vi "Protocole_son_preparatoire_2020.vi"() -> ()   [LabVIEW 2020]
uses:
  8c73e72c-2e4b-4090-9b5f-4dd0fd0f2149.vi
  bfbeb452-2a3a-4e65-bf29-1a1bdd43f38b.vi
  3aaf8e9c-9ac4-4c40-bc9e-b7ffdc0d35df.vi
  <vilib>/numeric/Random Number (Range) DBL.vi
  0129e9be-af5f-4d34-b4ce-d6aa148f68f5.vi
  2e48d409-a5b3-4865-bc36-115429370ffe.vi
  <vilib>/Analysis/1siggen.llb/General Gauss-Mod Sine.vi
  <vilib>/Analysis/NI_AALBase.lvlib
  <vilib>/measure/NI_MABase.lvlib
panel:
  in  "Control temps bruit 2":cluster{"Fs":dbl, "#s":dbl}={"Fs"=1000.0, "#s"=1000.0} {"Fs" format="%.2p"}
  in  "Control temps bruit":cluster{"Fs":dbl, "#s":dbl}={"Fs"=1000.0, "#s"=1000.0} {"Fs" format="%.2p"}
  in  "Nom du fichier":string="Test_"
  out "Barre de progression":dbl(slide) scale=0.0..100.0
  in  "?":enum32{"Temps", "Numérique "}(tab)
  in  "Temps d'attente entre chaque sons /s":dbl=2.0
  in  "Plus ou moins /s":dbl=1.0
  in  "Différence entre chaque fréquence /Hz":dbl=100.0
  in  "Fréquence min /Hz":dbl=440.0
  in  "Nombre de répétition d'opération":dbl=1.0
  in  "Nombre de sons":dbl=3.0
  in  "Amplitude min /V":dbl=0.5
  in  "Différence entre chaque amplitude /V":dbl=0.2
  in  "Lieu du fichier":path=path "D:/Labview/Stage/LabVIEW 2020/Programmes_utilisables/Protocoles_enregistrement_ampli/Protocole_son_preparatoire_2020/Donnees" caption="Filename"
  in  "?":bool
  # "Pas touché"
  # "Protocole :"
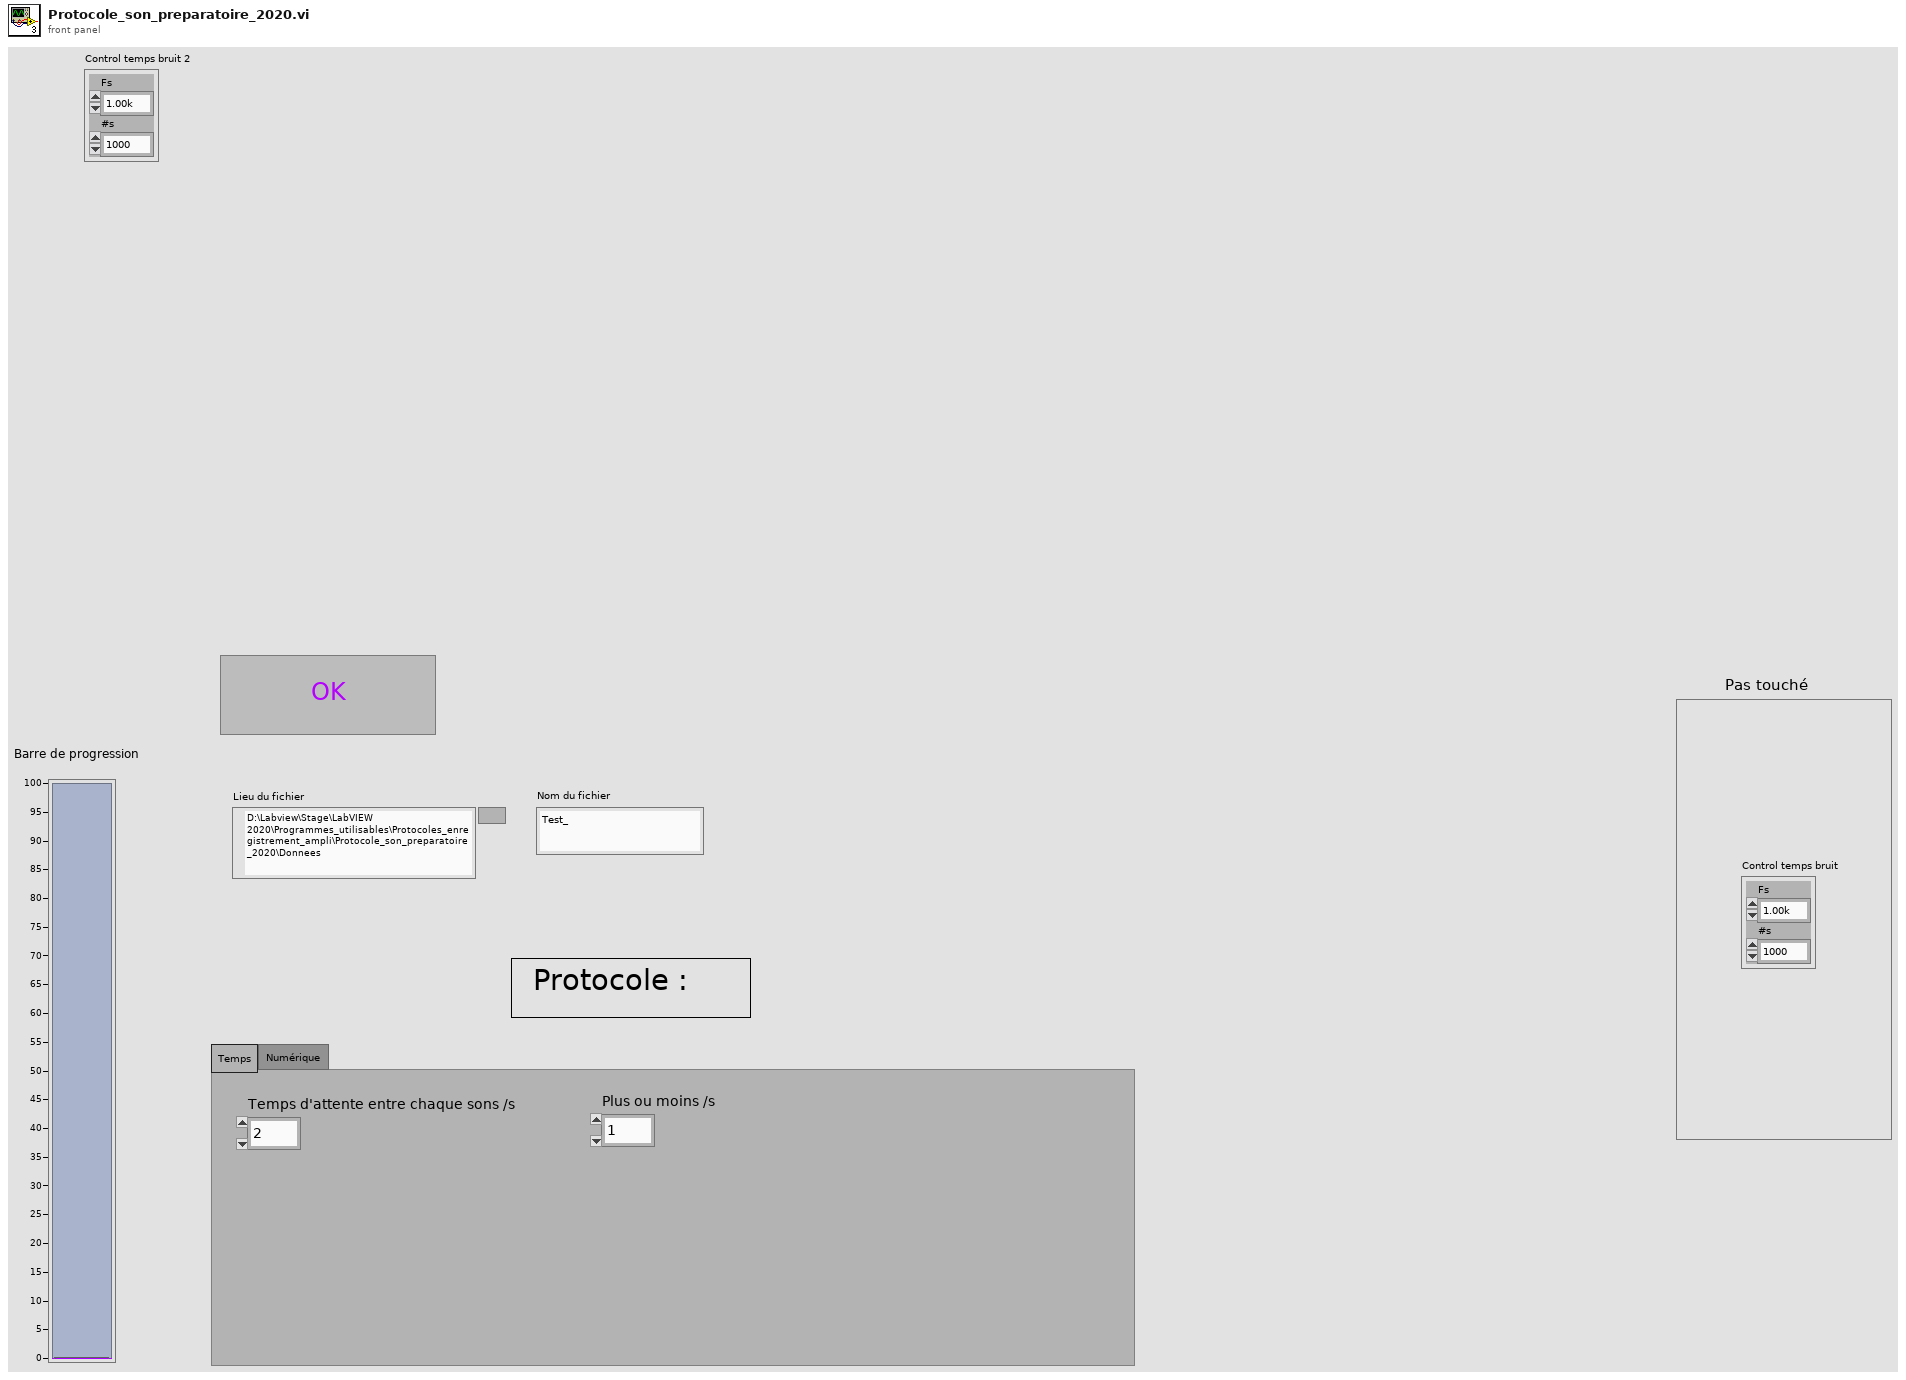
[diagram p1: front panel]
types:
  T1 = enum16{"open", "open or create", "create or replace", "create", "open (read-only)"}
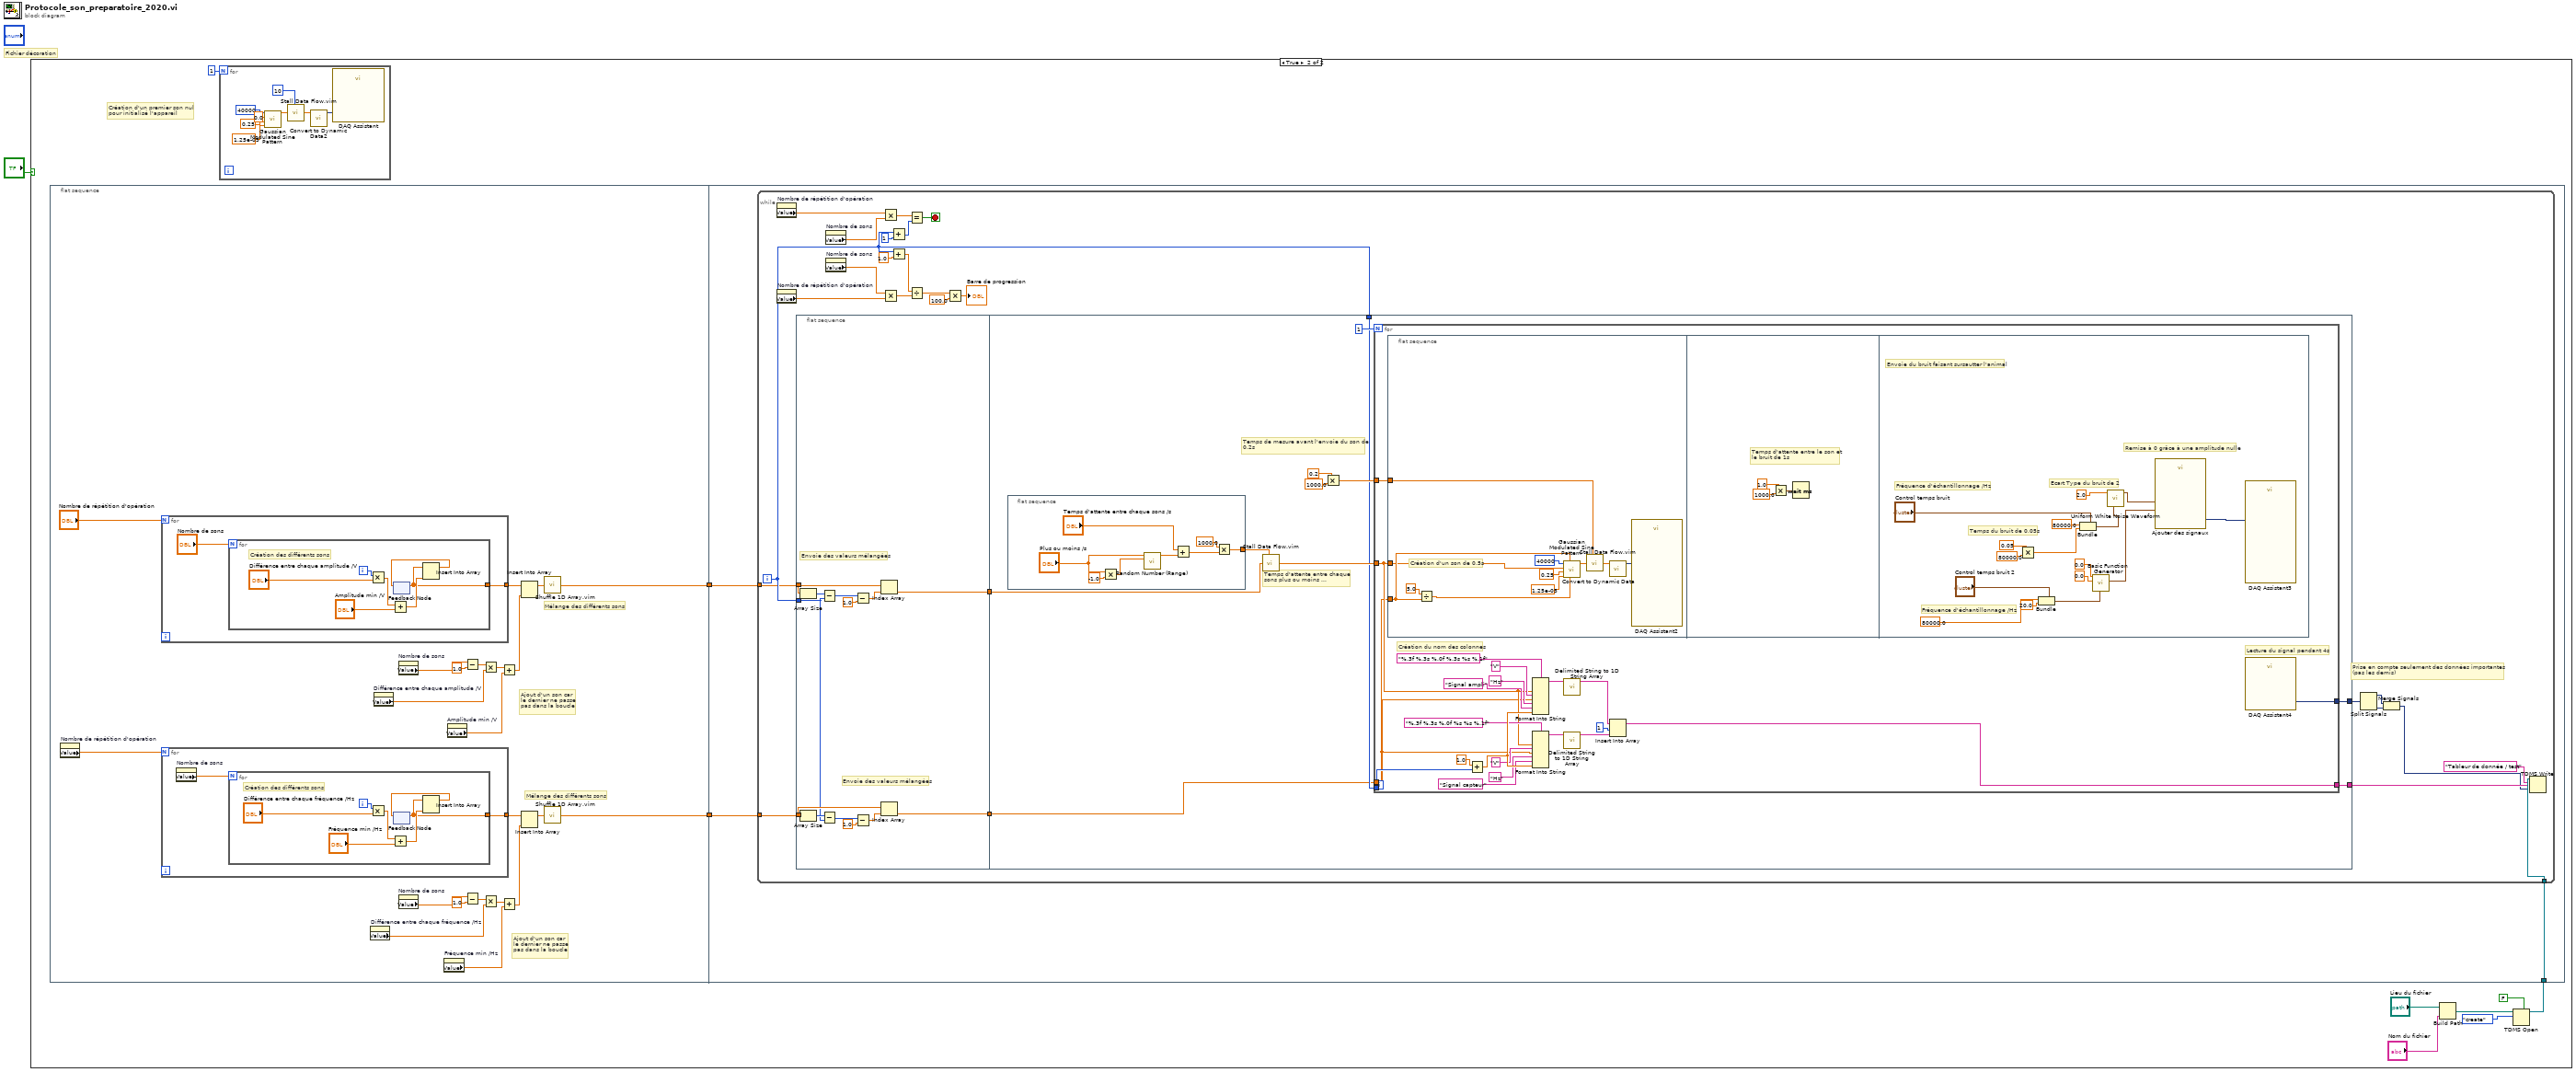
[diagram p0: block diagram]
diagram:
  # "Fichier décoration"
  n1 = case shown="True" "?" {
    frame False {
    }
    frame True {
      # "Création d'un premier son nul\npour initialisé l'appareil"
      n2 = flat-sequence {
        tunnel: [w31] -> w10
        tunnel: [w19] -> w3
        tunnel: w10 -> [w61]
        tunnel: w9 -> [w60]
        tunnel: w3 -> [w59]
        frame #0 {
          # "Mélange des différents sons"
          # "Ajout d'un son car \nle dernier ne passe \npas dans la boucle"
          # "Mélange des différents sons"
          # "Ajout d'un son car \nle dernier ne passe \npas dans la boucle"
          n3 = property on="Nombre de répétition d'opération" class="DigNum (strict)"() -> ("Value"=w23:dbl)  [unwired: 2 in, 2 out]
          n4 = for {
            N: "Nombre de répétition d'opération" -> [_]
            tunnel: [w50] -> w30
            n5 = for {
              N: "Nombre de sons" -> [_]
              tunnel: [w53] -> w50
              i -> [w57]
              # "Création des différents sons"
              n6 = Multiply(x=w57, y="Différence entre chaque amplitude /V") -> (x*y=w58:dbl)
              n7 = Add(x=w58, y="Amplitude min /V") -> (x+y=w54:dbl)
              n8 = feedback #1() -> (w53:dbl[])  [unwired: 1 in]
              n9 = Insert Into Array(array=w53, new element=w54) -> (w52:dbl[])  [unwired: 1 in]
              n10 = feedback-in #1(w52) -> ()
            }
          }
          n11 = for {
            N: w23 -> [_]
            tunnel: [w42] -> w24
            n12 = property on="Nombre de sons" class="DigNum (strict)"() -> ("Value"=w41:dbl)  [unwired: 2 in, 2 out]
            n13 = for {
              N: w41 -> [_]
              tunnel: [w46] -> w42
              i -> [w48]
              # "Création des différents sons"
              n14 = Multiply(x=w48, y="Différence entre chaque fréquence /Hz") -> (x*y=w49:dbl)
              n15 = Add(x=w49, y="Fréquence min /Hz") -> (x+y=w47:dbl)
              n16 = feedback #2() -> (w46:dbl[])  [unwired: 1 in]
              n17 = Insert Into Array(array=w46, new element=w47) -> (w45:dbl[])  [unwired: 1 in]
              n18 = feedback-in #2(w45) -> ()
            }
          }
          n19 = property on="Différence entre chaque fréquence /Hz" class="DigNum (strict)"() -> ("Value"=w21:dbl)  [unwired: 2 in, 2 out]
          n20 = property on="Différence entre chaque amplitude /V" class="DigNum (strict)"() -> ("Value"=w37:dbl)  [unwired: 2 in, 2 out]
          n21 = property on="Nombre de sons" class="DigNum (strict)"() -> ("Value"=w34:dbl)  [unwired: 2 in, 2 out]
          n22 = property on="Nombre de sons" class="DigNum (strict)"() -> ("Value"=w22:dbl)  [unwired: 2 in, 2 out]
          n23 = property on="Fréquence min /Hz" class="DigNum (strict)"() -> ("Value"=w20:dbl)  [unwired: 2 in, 2 out]
          n24 = property on="Amplitude min /V" class="DigNum (strict)"() -> ("Value"=w35:dbl)  [unwired: 2 in, 2 out]
          n25 = Subtract(x=w34, y=1.0) -> (x-y=w32:dbl)
          n26 = Subtract(x=w22, y=1.0) -> (x-y=w25:dbl)
          n27 = Multiply(x=w32, y=w37) -> (x*y=w36:dbl)
          n28 = Multiply(x=w25, y=w21) -> (x*y=w27:dbl)
          n29 = Add(x=w36, y=w35) -> (x+y=w39:dbl)
          n30 = Add(x=w27, y=w20) -> (x+y=w29:dbl)
          n31 = Insert Into Array(array=w30, new element=w39) -> (w38:dbl[])  [unwired: 1 in]
          n32 = Insert Into Array(array=w24, new element=w29) -> (w28:dbl[])  [unwired: 1 in]
          n33 = call "Shuffle 1D Array.vim"("array"=w38) -> ("shuffled array"=w31:dbl[])  [unwired: 4 in]
          n34 = call "Shuffle 1D Array.vim"("array"=w28) -> ("shuffled array"=w19:dbl[])  [unwired: 4 in]
        }
        frame #1 {
          n35 = while {
            tunnel: w61 -> [w68]
            tunnel: w60 -> [w73]
            tunnel: w59 -> [w67]
            i -> [w70]
            stop <- w84 stop-if-true
            # "Prise en compte seulement des données importantes \n(pas les demis)"
            n36 = property on="Nombre de répétition d'opération" class="DigNum (strict)"() -> ("Value"=w87:dbl)  [unwired: 2 in, 2 out]
            n37 = property on="Nombre de répétition d'opération" class="DigNum (strict)"() -> ("Value"=w80:dbl)  [unwired: 2 in, 2 out]
            n38 = flat-sequence {
              tunnel: w68 -> [w100]
              tunnel: w70 -> [w88]
              tunnel: [w98] -> w83
              tunnel: w67 -> [w90]
              tunnel: [w89] -> w66
              tunnel: w83 -> [w110]
              tunnel: [w103] -> w65
              tunnel: [w104] -> w71
              tunnel: w70 -> [w105]
              tunnel: w66 -> [w102]
              frame #0 {
                # "Envoie des valeurs mélangées"
                # "Envoie des valeurs mélangées"
                n39 = Array Size(array=w100) -> (size(s)=w99:i32)
                n40 = Array Size(array=w90) -> (size(s)=w94:i32)
                n41 = Subtract(x=w99, y=w88) -> (x-y=w96:i32)
                n42 = Subtract(x=w94, y=w88) -> (x-y=w92:i32)
                n43 = Subtract(x=w96, y=1.0) -> (x-y=w95:dbl)
                n44 = Subtract(x=w92, y=1.0) -> (x-y=w91:dbl)
                n45 = Index Array(array=w100, index=w95) -> (element=w98:dbl)
                n46 = Index Array(array=w90, index=w91) -> (element=w89:dbl)
              }
              frame #1 {
                # "Temps de mesure avant l'envoie du son de \n0,2s"
                # "Temps d'attente entre chaque \nsons plus ou moins ..."
                n47 = flat-sequence {
                  tunnel: [w166] -> w109
                  frame #0 {
                    n48 = Multiply(x="Plus ou moins /s", y=-1.0) -> (x*y=w164:dbl)
                    n49 = call-poly <vilib>:"Random Number (Range).vi"("lower bound (0)"=w164, "upper bound (100)"="Plus ou moins /s") -> ("number"=w165:dbl)  [unwired: 9 in]
                    n50 = Add(x="Temps d'attente entre chaque sons /s", y=w165) -> (x+y=w170:dbl)
                    n51 = Multiply(x=1000.0, y=w170) -> (x*y=w166:dbl)
                  }
                }
                n52 = call "Stall Data Flow.vim"("value in"=w110, "milliseconds to wait"=w109) -> ("value out"=w106:dbl)  [unwired: 1 out]
                n53 = Multiply(x=0.2, y=1000.0) -> (x*y=w107:dbl)
                n54 = for {
                  N: 1 -> [_]
                  tunnel: w102 -> [w112]
                  tunnel: w106 -> [w113]
                  tunnel: w107 -> [w114]
                  tunnel: w105 -> [w127]
                  tunnel: [w116] -> w104
                  tunnel: [w115] -> w103
                  # "Création du nom des colonnes"
                  # "Lecture du signal pendant 4s"
                  n55 = flat-sequence {
                    tunnel: w114 -> [w135]
                    tunnel: w112 -> [w134]
                    tunnel: w113 -> [w133]
                    frame #0 {
                      # "Création d'un son de 0,5s"
                      n56 = Divide(x=5.0, y=w134) -> (x/y=w137:dbl)
                      n57 = call <vilib>:"Gaussian Modulated Sine Pattern.vi"("normalized bandwidth"=w137, "center frequency (Hz)"=w134, "delta t (s)"=1.25e-05, "delay (s)"=0.25, "amplitude"=w133, "samples"=40000) -> ("Gauss-Mod Sine Pattern"=w143:dbl[])  [unwired: 4 in, 1 out]
                      n58 = call "Stall Data Flow.vim"("value in"=w143, "milliseconds to wait"=w135) -> ("value out"=w142:dbl[])  [unwired: 1 out]
                      n59 = call "Convert to Dynamic Data"("Array"=w142) -> ("Dynamic Data Type"=w136:dynamicdata)  [unwired: 3 in]
                      n60 = call "DAQ Assistant2"("data"=w136) -> ()  [unwired: 17 in, 2 out]
                    }
                    frame #1 {
                      # "Temps d'attente entre le son et\nle bruit de 1s"
                      n61 = Multiply(x=1.0, y=1000.0) -> (x*y=w146:dbl)
                      n62 = Wait (ms)(milliseconds to wait=w146) -> ()  [unwired: 1 out]
                    }
                    frame #2 {
                      # "Ecart Type du bruit de 2"
                      # "Temps du bruit de 0,05s"
                      # "Remise à 0 grâce à une amplitude nulle"
                      # "Fréquence d'échantillonnage /Hz"
                      # "Envoie du bruit faisant sursautter l'animal"
                      # "Fréquence d'échantillonnage /Hz"
                      n63 = Multiply(x=0.05, y=80000.0) -> (x*y=w161:dbl)
                      n64 = Bundle(cluster="Control temps bruit 2", "Fs"=80000.0, "#s"=20.0) -> (w153:cluster{"Fs":dbl, "#s":dbl})
                      n65 = Bundle(cluster="Control temps bruit", "Fs"=80000.0, "#s"=w161) -> (w148:cluster{"Fs":dbl, "#s":dbl})
                      n66 = call <vilib>:"Basic Function Generator.vi"("sampling info"=w153, "amplitude"=0.0, "frequency"=0.0) -> ("signal out"=w158:waveform(dbl))  [unwired: 6 in, 2 out]
                      n67 = call <vilib>:"Uniform White Noise Waveform.vi"("sampling info"=w148, "amplitude"=2.0 ("standard deviation")) -> ("signal out"=w147:waveform(dbl))  [unwired: 8 in, 1 out]
                      n68 = call "Ajouter des signaux"("Input Signal B"=w158, "Input Signal A"=w147) -> ("Appended Signals"=w151:dynamicdata)  [unwired: 8 in, 1 out]
                      n69 = call "DAQ Assistant3"("data"=w151) -> ()  [unwired: 17 in, 2 out]
                    }
                  }
                  n70 = Add(x=1.0, y=w127) -> (x+y=w132:dbl)
                  n71 = Format Into String(format string="%.3f %.3s %.0f %.3s %s %.1f" ("chaîne de format"), w113, "V" ("entrée 2"), w112, "Hz" ("entrée 4"), "Signal ampli" ("entrée 2"), w132) -> (resulting string=w128:string)  [unwired: 2 in, 1 out]
                  n72 = Format Into String(format string="%.3f %.3s %.0f %s %s %.1f" ("chaîne de format"), w113, "V" ("entrée 2"), w112, "Hz" ("entrée 4"), "Signal capteur" ("entrée 2"), w132) -> (resulting string=w129:string)  [unwired: 2 in, 1 out]
                  n73 = call <vilib>:"Delimited String to 1D String Array.vi"("delimited string"=w128) -> ("string array"=w131:string[])  [unwired: 10 in]
                  n74 = call <vilib>:"Delimited String to 1D String Array.vi"("delimited string"=w129) -> ("string array"=w130:string[])  [unwired: 10 in]
                  n75 = Insert Into Array(array=w131, index=1 ("indice"), new element=w130) -> (w116:string[])
                  n76 = call "DAQ Assistant4"() -> ("data"=w115:dynamicdata)  [unwired: 17 in, 2 out]
                }
              }
            }
            n77 = property on="Nombre de sons" class="DigNum (strict)"() -> ("Value"=w86:dbl)  [unwired: 2 in, 2 out]
            n78 = property on="Nombre de sons" class="DigNum (strict)"() -> ("Value"=w79:dbl)  [unwired: 2 in, 2 out]
            n79 = Multiply(x=w87, y=w86) -> (x*y=w85:dbl)
            n80 = Multiply(x=w79, y=w80) -> (x*y=w78:dbl)
            n81 = Add(x=w70, y=1) -> (x+y=w81:i32)
            n82 = Add(x=w70, y=1.0) -> (x+y=w74:dbl)
            n83 = Equal?(x=w85, y=w81) -> (x = y?=w84:bool)
            n84 = Divide(x=w74, y=w78) -> (x/y=w76:dbl)
            n85 = Multiply(x=w76, y=100.0) -> (x*y=→"Barre de progression":dbl)
            n86 = Split Signals(w65) -> (w64:dynamicdata, w63:dynamicdata)  [unwired: 4 in, 2 out]
            n87 = Merge Signals(w64, w63) -> (w62:dynamicdata)
            n88 = TDMS Write(0:w73, 5:"Tableur de donnée / test" ("nom du groupe en entrée (Sans titre)"), 7:w71, 9:w62) -> ()  [unwired: 2 in, 4 out]
          }
        }
      }
      n89 = for {
        N: 1 -> [_]
        n90 = call <vilib>:"Gaussian Modulated Sine Pattern.vi"("delta t (s)"=1.25e-05, "delay (s)"=0.25, "amplitude"=0.0, "samples"=40000) -> ("Gauss-Mod Sine Pattern"=w18:dbl[])  [unwired: 6 in, 1 out]
        n91 = call "Stall Data Flow.vim"("value in"=w18, "milliseconds to wait"=u32 10) -> ("value out"=w17:dbl[])  [unwired: 1 out]
        n92 = call "Convert to Dynamic Data2"("Array"=w17) -> ("Dynamic Data Type"=w13:dynamicdata)  [unwired: 3 in]
        n93 = call "DAQ Assistant"("data"=w13) -> ()  [unwired: 17 in, 2 out]
      }
      n94 = Build Path(base path="Lieu du fichier", name or relative path="Nom du fichier") -> (appended path=w6:path)
      n95 = TDMS Open(5:FALSE ("créer un fichier index ? (V)"), 10:T1."create" ("opération (0 : open)"), 11:w6) -> (3:w9:refnum<k34>)  [unwired: 4 in, 1 out]
    }
  }
